vi "MGI Set Front Panel Title.vi"(7 "Error In":errorcluster, 9 "Front Panel Window:Title":string, 10 "VI Reference In (Caller)":refnum<vi>) -> (0 "Error Out":errorcluster, 3 "VI Reference Out":refnum<vi>)   [LabVIEW 2016]
doc: "Sets the Front Panel Title of the referenced VI.\n\nAuthored by Robert C. Mortensen\nsupport@mooregoodideas.com\nwww.mooregoodideas.com\n\nCopyright (c) 2010, Moore Good Ideas, Inc.\n\nAll rights reserved.\n\nRedistribution and use in source and binary forms, with or without modification, are permitted provided that the following conditions are met:\n\n * Redistributions of source code must retain the above copyright notice, this list of conditions and the following disclaimer.\n * Redistributions in binary form must reproduce the above copyright notice, this list of conditions and the following disclaimer in the documentation and/or other materials provided with the distribution.\n * Neither the name of Moore Good Ideas, Inc. nor the names of its contributors may be used to endorse or promote products derived from this software without specific prior written permission.\n\nTHIS SOFTWARE IS PROVIDED BY THE COPYRIGHT HOLDERS AND CONTRIBUTORS \"AS IS\" AND ANY EXPRESS OR IMPLIED WARRANTIES, INCLUDING, BUT NOT LIMITED TO, THE IMPLIED WARRANTIES OF MERCHANTABILITY AND FITNESS FOR A PARTICULAR PURPOSE ARE DISCLAIMED. IN NO EVENT SHALL THE COPYRIGHT OWNER OR CONTRIBUTORS BE LIABLE FOR ANY DIRECT, INDIRECT, INCIDENTAL, SPECIAL, EXEMPLARY, OR CONSEQUENTIAL DAMAGES (INCLUDING, BUT NOT LIMITED TO, PROCUREMENT OF SUBSTITUTE GOODS OR SERVICES; LOSS OF USE, DATA, OR PROFITS; OR BUSINESS INTERRUPTION) HOWEVER CAUSED AND ON ANY THEORY OF LIABILITY, WHETHER IN CONTRACT, STRICT LIABILITY, OR TORT (INCLUDING NEGLIGENCE OR OTHERWISE) ARISING IN ANY WAY OUT OF THE USE OF THIS SOFTWARE, EVEN IF ADVISED OF THE POSSIBILITY OF SUCH DAMAGE."
uses:
  <userlib>/_MGI/Application Control/MGI VI Reference/MGI Caller's VI Reference.vi
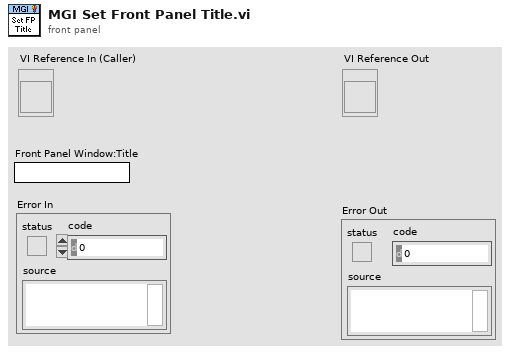
[diagram p1: front panel]
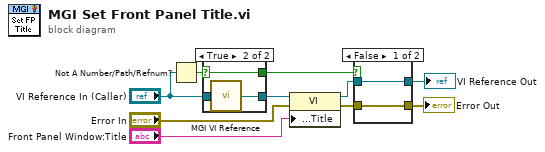
[diagram p0: block diagram]
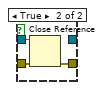
[diagram p2: hidden frame]
diagram:
  n1 = Not A Number/Path/Refnum?(number/path/refnum="VI Reference In (Caller)") -> (NaN/Path/Refnum?=w5:bool)
  n2 = case shown="True" w5 {
    selector: w5 -> [_ w12]
    tunnel: [w11 w13] -> w4
    tunnel: "VI Reference In (Caller)" -> [w11 _]
    tunnel: [_ w12] -> w2
    frame False {
    }
    frame True {
      n3 = call-poly <userlib>:"MGI VI Reference.vi"() -> ("Caller's VI Reference"=w13:refnum<vi>)  [unwired: 1 in]
    }
  }
  n4 = property class="VI"(reference=w4, error in="Error In", "Front Panel Window:Title"="Front Panel Window:Title") -> (reference out=w8:refnum<vi>, error out=w9:errorcluster)
  n5 = case shown="False" w2 {
    tunnel: w9 -> [w15 w18]
    tunnel: w8 -> [w14 w17]
    tunnel: [w15 w16] -> w7
    tunnel: [w14 _] -> w1
    frame False {
    }
    frame True {
      n6 = Close Reference(reference=w17, error in (no error)=w18) -> (error out=w16:errorcluster)
    }
  }
  "Error Out" <- w7
  "VI Reference Out" <- w1
